vi "publishLargeFileObjectAvailable.vi"(8 "error in (no error)":errorcluster, 11 "Model in":refnum<class "Model.lvclass">) -> (0 "error out":errorcluster, 3 "Model out":refnum<class "Model.lvclass">)   [LabVIEW 2016, in "Model.lvclass"]
uses:
  Model.lvclass
  Typedefs/PubDataSignals.ctl
  ts_sallv_FiberSpectrograph/DataTypes/logevent_largeFileObjectAvailable.ctl
  Model.lvclass/Model.ctl
  CFitsIO/CFitsIO.lvclass
  Typedefs/FiberSpectrographTypedefs.lvlib
  ts_sallv_FiberSpectrograph/SALLV_FiberSpectrograph.lvlib
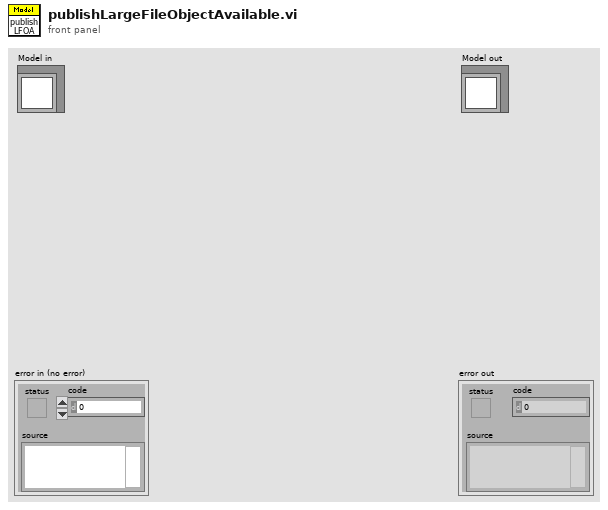
[diagram p1: front panel]
types:
  T1 = typedef "SALLV_FiberSpectrograph.lvlib/logevent_largeFileObjectAvailable.ctl" = cluster{"url":string, "generator":string, "version":sgl, "byteSize":i32, "checkSum":string, "mimeType":string, "id":string, "priority":i32}
  T2 = typedef "FiberSpectrographTypedefs.lvlib/PubDataSignals.ctl" = enum16{"DetailedState", "ErrorCode", "Heartbeat", "LoopTime_ms", "LoopTimeOutOfRange", "RejectedCommand", "SummaryState", "Timestamp", "SettingVersions", "AppliedSettingsMatchStart", "TimeOut", "MeasuredSpectrum", "LargeFileObjectAvailable"}
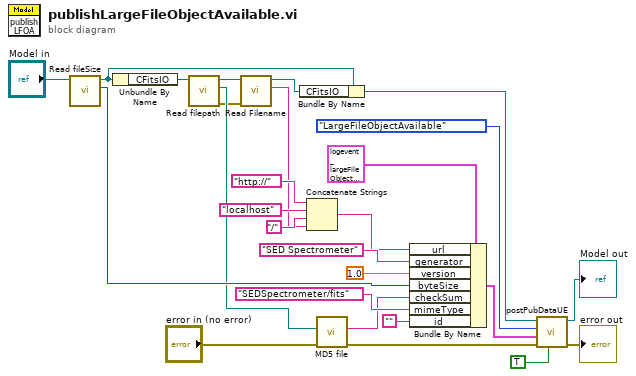
[diagram p0: block diagram]
diagram:
  n1 = call-dynamic "Read fileSize.vi"("Model in"="Model in") -> ("file size (in bytes)"=w16:i64, "Model out"=w6:refnum<class "Model.lvclass">)  [unwired: 8 in, 1 out]
  n2 = Unbundle By Name(w6) -> ("CFitsIO"=w19:refnum<class "CFitsIO.lvclass">)
  n3 = call-dynamic "Read filepath.vi"("CFitsIO in"=w19) -> ("error out"=w8:errorcluster, "Filepath"=w13:path, "CFitsIO out"=w9:refnum<class "CFitsIO.lvclass">)  [unwired: 8 in]
  n4 = call-dynamic "Read Filename.vi"("error in (no error)"=w8, "CFitsIO in"=w9) -> ("Filename"=w1:string, "CFitsIO out"=w7:refnum<class "CFitsIO.lvclass">)  [unwired: 7 in, 1 out]
  n5 = Bundle By Name(cluster=w6, "CFitsIO"=w7) -> (w5:refnum<class "Model.lvclass">)
  n6 = Concatenate Strings("http://" ("string"), "localhost" ("string"), "/" ("string"), w1) -> (w18:string)
  n7 = call "MD5 file.vi"("error in (no error)"="error in (no error)", "Path"=w13) -> ("error out"=w10:errorcluster, "MD5 message-digest"=w12:string)  [unwired: 8 in]
  n8 = Bundle By Name(cluster=T1 {"url"="", "generator"="                                                                                                                                                                                                                                                                ", "version"=0.0, "byteSize"=0, "checkSum"="                                ", "mimeType"="                                ", "id"="                                ", "priority"=0} ("logevent_LargeFileObjectAvailable"), "url"=w18, "generator"="SED Spectrometer" ("Generator"), "version"=sgl 1.0 ("Version"), "byteSize"=w16, "checkSum"=w12, "mimeType"="SEDSpectrometer/fits" ("Mime_Type"), "id"="" ("ID")) -> (w22:T1)
  n9 = call "postPubDataUE.vi"("newValue (T)"=TRUE, "error in (no error)"=w10, "value"=w22, "pubDataSV"=PubDataSignals."LargeFileObjectAvailable", "Model in"=w5) -> ("error out"=→"error out":errorcluster, "Model out"=→"Model out":refnum<class "Model.lvclass">)  [unwired: 5 in]
